vi "Read Device.lvclass.vi"(8 "Error in":errorcluster, 11 "Test in":refnum<class "Test.lvclass">) -> (0 "Error out":errorcluster, 2 "Device.lvclass":refnum<class "Device.lvclass">, 3 "Test out":refnum<class "Test.lvclass">)   [LabVIEW 2020, in "Test.lvclass"]
uses:
  Test.lvclass
  Class/INL DNL Test/Device/Parent/Device.lvclass
  Test.lvclass/Test.ctl
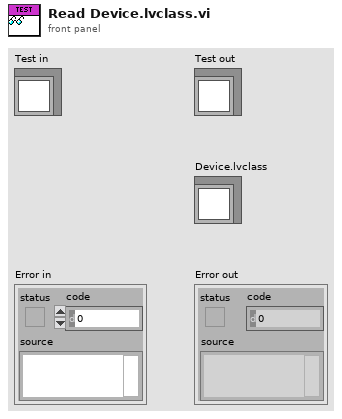
[diagram p1: front panel]
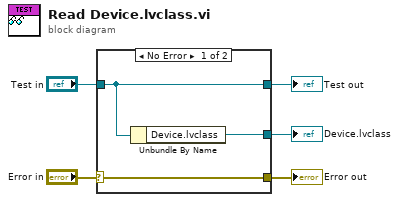
[diagram p0: block diagram]
diagram:
  n1 = case shown="No Error" "Error in" {
    selector: "Error in" -> [w8 w9]
    tunnel: [w8 w9] -> w4
    tunnel: [w7 w10] -> w2
    tunnel: "Test in" -> [w7 w10]
    tunnel: [w6 _] -> w1
    frame No Error {
      n2 = Unbundle By Name(w7) -> ("Device.lvclass"=w6:refnum<class "Device.lvclass">)
    }
    frame Error {
    }
  }
  "Error out" <- w4
  "Test out" <- w2
  "Device.lvclass" <- w1
